vi "Delete Directory.vi"(6 "timeout (ms)":i32=30000, 8 "error in":errorcluster, 10 "path":string, 11 "session in":refnum<class "Session.lvclass">) -> (0 "error out":errorcluster, 3 "session out":refnum<class "Session.lvclass">)   [LabVIEW 2020, in "NI_SFTP.lvlib"]
doc: "Deletes a remote directory. Use <b>Delete File</b> to delete files."
uses:
  <vilib>/net/SFTP/NI_SFTP.lvlib
  <vilib>/net/SFTP/Session/Session.lvclass
  <vilib>/Utility/Deadline/NI_Deadline.lvlib
  <vilib>/net/SFTP/API/Support/Command/SSH_FXP_RMDIR/SSH_FXP_RMDIR.lvclass
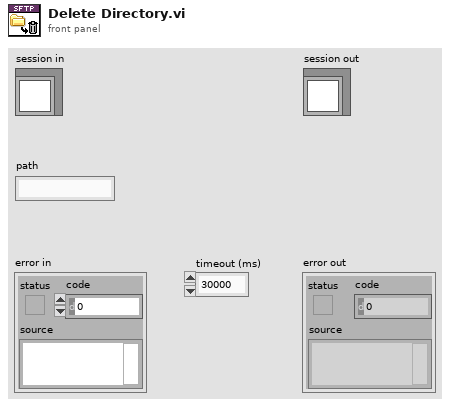
[diagram p1: front panel]
types:
  T1 = typedef "NI_Deadline.lvlib/Deadline.ctl" = cluster{"mode":T2, "deadline (ms)":u32}
  T2 = typedef "NI_Deadline.lvlib/Mode.ctl" = enum16{"Relative", "Use deadline", "Wait forever", "Nonblocking", "N/A"}
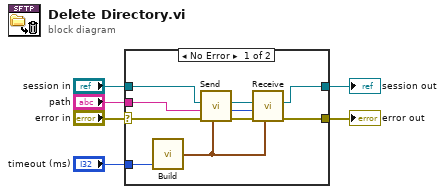
[diagram p0: block diagram]
diagram:
  n1 = case shown="No Error" "error in" {
    selector: "error in" -> [w12 w18]
    tunnel: [w11 w18] -> w5
    tunnel: [w7 w17] -> w3
    tunnel: "session in" -> [w10 w17]
    tunnel: "path" -> [w9 _]
    tunnel: "timeout (ms)" -> [w16 _]
    frame No Error {
      n2 = call <vilib>:"Build.vi"("timeout (ms)"=w16) -> ("Deadline out"=w13:T1)  [unwired: 2 in]
      n3 = call <vilib>:"Send.vi"("Timeout"=w13, "error in (no error)"=w12, "path"=w9, "session in"=w10) -> ("error out"=w15:errorcluster, "request id"=w8:u32, "session out"=w14:refnum<class "Session.lvclass">)  [unwired: 4 in, 1 out]
      n4 = call <vilib>:"Receive.vi"("Timeout"=w13, "error in (no error)"=w15, "request id"=w8, "session in"=w14) -> ("error out"=w11:errorcluster, "session out"=w7:refnum<class "Session.lvclass">)  [unwired: 4 in, 2 out]
    }
    frame Error {
    }
  }
  "error out" <- w5
  "session out" <- w3
